vi "Colorize.vi"(8 "error in (no error)":errorcluster, 9 "Tag":string, 10 "Type Descriptor Enum":T1 format="%.0x", 11 "VariantTree in":refnum<class "Failures_VariantTree__VP.lvclass">) -> (0 "error out":errorcluster, 3 "VariantTree out":refnum<class "Failures_VariantTree__VP.lvclass">)   [LabVIEW 2013, in "Failures_VariantTree__VP.lvclass"]
uses:
  Failures_VariantTree__VP.lvclass
  <userlib>/_OpenG.lib/lvdata/lvdata.llb/Type Descriptor Enumeration__ogtk.ctl
  Failures_VariantTree__VP.lvclass/Failures_VariantTree__VP.ctl
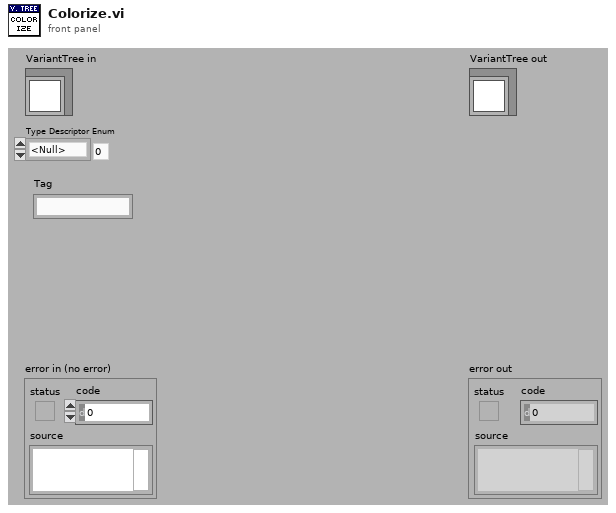
[diagram p1: front panel]
types:
  T1 = typedef "Type Descriptor Enumeration__ogtk.ctl" = enum8{"<Null>", "I8", "I16", "I32", "I64", "U8", "U16", "U32", "U64", "SGL", "DBL", "EXT", "CSG", "CDB", "CXT", "0x0F", "0x10", "0x11", "0x12", "0x13", "0x14", "Enum U8", "Enum U16", "Enum U32", "Enum U64", "SGL PQ", "DBL PQ", "EXT PQ", "CSG PQ", "CDB PQ", "CXT PQ", "0x1F", "0x20", "Boolean", "0x22", "0x23", "0x24", "0x25", "0x26", "0x27", "0x28", "0x29", "0x2A", "0x2B", "0x2C", "0x2D", "0x2E", "0x2F", "String", "0x31", "Path", "Pict", "0x34", "0x35", "0x36", "DAQ", "0x38", "0x39", "0x3A", "0x3B", "0x3C", "0x3D", "0x3E", "0x3F", "Array", "0x41", "0x42", "0x43", "0x44", "0x45", "0x46", "0x47", "0x48", "0x49", "0x4A", "0x4B", "0x4C", "0x4D", "0x4E", "0x4F", "Cluster", "0x51", "0x52", "Variant", "Waveform", "0x55", "0x56", "0x57", "0x58", "0x59", "0x5A", "0x5B", "0x5C", "0x5D", "0x5E", "0x5F", "0x60", "0x61", "0x62", "0x63", "0x64", "0x65", "0x66", "0x67", "0x68", "0x69", "0x6A", "0x6B", "0x6C", "0x6D", "0x6E", "0x6F", "Refnum"}
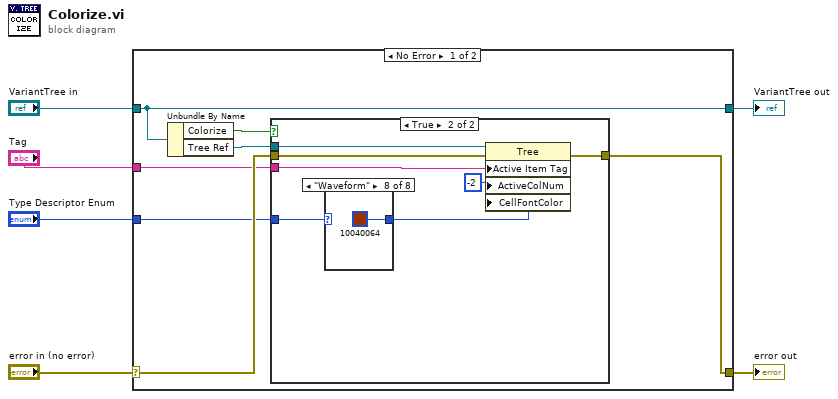
[diagram p0: block diagram]
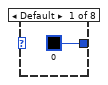
[diagram p3: hidden frame]
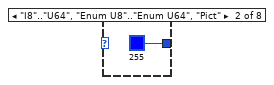
[diagram p4: hidden frame]
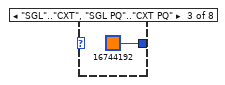
[diagram p5: hidden frame]
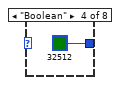
[diagram p6: hidden frame]
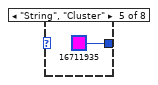
[diagram p7: hidden frame]
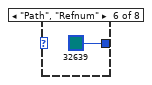
[diagram p8: hidden frame]
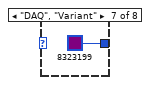
[diagram p9: hidden frame]
diagram:
  n1 = case shown="No Error" "error in (no error)" {
    selector: "error in (no error)" -> [w10 w31]
    tunnel: [w7 w31] -> w5
    tunnel: [w13 w30] -> w3
    tunnel: "VariantTree in" -> [w13 w30]
    tunnel: "Type Descriptor Enum" -> [w9 _]
    tunnel: "Tag" -> [w8 _]
    frame No Error {
      n2 = Unbundle By Name(w13) -> ("Colorize"=w12:bool, "Tree Ref"=w11:refnum<vi>)
      n3 = case shown="True" w12 {
        tunnel: w11 -> [_ w20]
        tunnel: w10 -> [w14 w19]
        tunnel: w9 -> [_ w21]
        tunnel: w8 -> [_ w18]
        tunnel: [w14 w15] -> w7
        frame False {
        }
        frame True {
          n4 = case shown="\"Waveform\"" w21 {
            tunnel: [u32 0 u32 255 u32 16744192 u32 32512 u32 16711935 u32 32639 u32 8323199 u32 10040064] -> w16
            frame Default {
            }
            frame "I8".."U64", "Enum U8".."Enum U64", "Pict" {
            }
            frame "SGL".."CXT", "SGL PQ".."CXT PQ" {
            }
            frame "Boolean" {
            }
            frame "String", "Cluster" {
            }
            frame "Path", "Refnum" {
            }
            frame "DAQ", "Variant" {
            }
            frame "Waveform" {
            }
          }
          n5 = property class="Tree"(reference=w20, error in=w19, "Active Item Tag"=w18, "ActiveColNum"=-2 ("Active Cell:Active Column Number"), "CellFontColor"=w16) -> (error out=w15:errorcluster)  [unwired: 1 out]
        }
      }
    }
    frame Error {
    }
  }
  "error out" <- w5
  "VariantTree out" <- w3
